vi "merFISH_hybridization_valve.vi"(1 "queue valve":refnum<queue>, 2 "error in":errorcluster, 3 "New position":i32, 4 "Valve H":u8(knob)=1 min=1 max=22 scale=1.0..22.0) -> (0 "error out":errorcluster)   [LabVIEW 2015]
uses:
  CONTROLS/Q_VALVE_element.ctl
  GLOBAL/Global_ABORT.vi
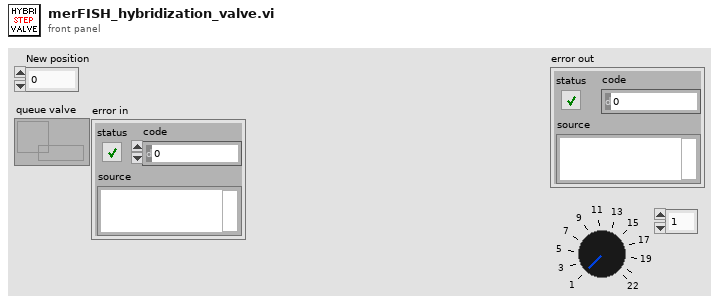
[diagram p1: front panel]
types:
  T1 = typedef "Q_VALVE_element.ctl" = cluster{"variant":variant, "Instruction":enum16{"VALVE_idle", "VALVE_initialize", "VALVE_error", "VALVE_security_stop", "VALVE_change_position", "VALVE_two_way_valves", "VALVE_init_merFISH", "VALVE_stop"}}
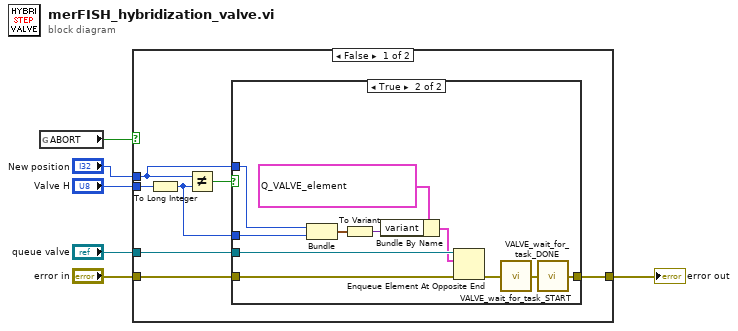
[diagram p0: block diagram]
diagram:
  n1 = global read "Global_ABORT.vi" "ABORT"() -> (w2:bool)
  n2 = case shown="False" w2 {
    tunnel: "queue valve" -> [w13 _]
    tunnel: "error in" -> [w12 w26]
    tunnel: "Valve H" -> [w10 _]
    tunnel: [w9 w26] -> w4
    tunnel: "New position" -> [w8 _]
    frame False {
      n3 = To Long Integer(number=w10) -> (32bit integer=w7:i32)
      n4 = Not Equal?(x=w8, y=w7) -> (x != y?=w11:bool)
      n5 = case shown="True" w11 {
        tunnel: w13 -> [_ w25]
        tunnel: w12 -> [w14 w24]
        tunnel: [w14 w18] -> w9
        tunnel: w7 -> [_ w17]
        tunnel: w8 -> [_ w15]
        frame False {
        }
        frame True {
          n6 = Bundle("New position"=w15, w17) -> (w16:cluster{"New position":i32, i32})  [unwired: 1 in]
          n7 = To Variant(anything=w16) -> (Variant=w22:variant)
          n8 = Bundle By Name(cluster=T1 {"variant"=variant, "Instruction"=enum."VALVE_change_position"} ("element"), "variant"=w22) -> (w21:T1)
          n9 = Enqueue Element At Opposite End(queue=w25, element=w21, error in (no error)=w24) -> (error out=w20:errorcluster)  [unwired: 1 in, 2 out]
          n10 = call "VALVE_wait_for_task_START.vi"("error in"=w20) -> ("error out"=w19:errorcluster)
          n11 = call "VALVE_wait_for_task_DONE.vi"("error in"=w19) -> ("error out"=w18:errorcluster)
        }
      }
    }
    frame True {
    }
  }
  "error out" <- w4
